vi "PVCAM_GetParam.vi"(8 "error in (no error)":errorcluster, 9 "param_attrib":T1(ring), 10 "param_id":u32, 11 "hCam":i16) -> (0 "error out":errorcluster, 2 "return type":i16, 3 "param_value":i16)   [LabVIEW 2021]
uses:
  pvcam64.dll
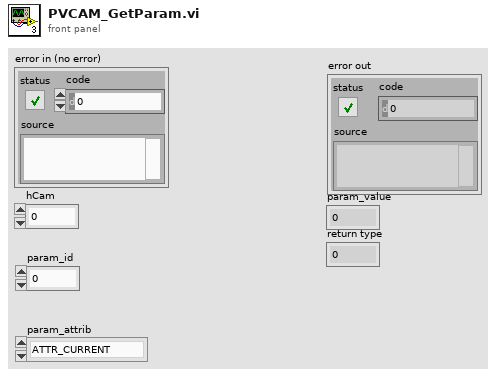
[diagram p1: front panel]
types:
  T1 = enum16{"ATTR_CURRENT", "ATTR_COUNT", "ATTR_TYPE", "ATTR_MIN", "ATTR_MAX", "ATTR_DEFAULT", "ATTR_INCREMENT", "ATTR_ACCESS", "ATTR_AVAIL"}
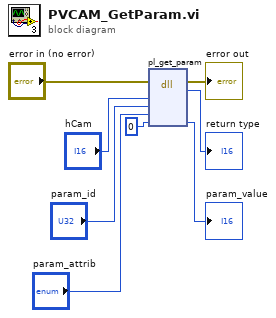
[diagram p0: block diagram]
diagram:
  n1 = dll-call lib="pvcam64.dll" fn="pl_get_param"(error in="error in (no error)", "hCam"="hCam", "param_id"="param_id", "param_attrib"="param_attrib", "param_value"=i16 0) -> (error out=→"error out":errorcluster, "return type"=→"return type":i16, "param_value"=→"param_value":i16)  [unwired: 5 in, 1 out]
